vi "example test.vi"() -> ()   [LabVIEW 2013, in "io plugin tests.lvlib"]
uses:
  io plugin tests.lvlib
  module/configuration/tag bus configurable plugin module configuration.lvclass
  <vilib>/NI/Tag Bus Module Framework/channel/channel classification.ctl
  <vilib>/NI/Tag Bus/tag/Data Type.ctl
  module/execution/tag bus configurable plugin module.lvclass
  <vilib>/NI/Tag Bus/dictionary/data dictionary.lvclass/data dictionary.ctl
  <vilib>/NI/Tag Bus/dictionary/lookup polymorphs/locate double.vi
  <vilib>/NI/Tag Bus/table/data polymorphs/write one/write Double.vi
  <vilib>/NI/Tag Bus/table/data polymorphs/read one/read Double.vi
  <vilib>/NI/Tag Bus/dictionary/search/find data index.vi
  <vilib>/NI/Tag Bus/dictionary/search/search string list.vi
  <vilib>/NI/Tag Bus/dictionary/tag not found.vi
  <vilib>/NI/Tag Bus Module Framework/channel/TBM channel.lvclass
  <vilib>/NI/Tag Bus/tag/tag descriptor.lvclass
  <vilib>/NI/Tag Bus/dictionary/data dictionary.lvclass
  <vilib>/NI/Tag Bus/table/data table.lvlib
panel:
  out "final error":errorcluster
  out "output error":errorcluster
  out "input error":errorcluster
  out "output lookup error":errorcluster
  out "no data written":bool
  out "input lookup error":errorcluster
  out "init error":errorcluster
  out "correct execution settings":bool
  out "serialization problem":errorcluster
  out "invalid configuration":errorcluster
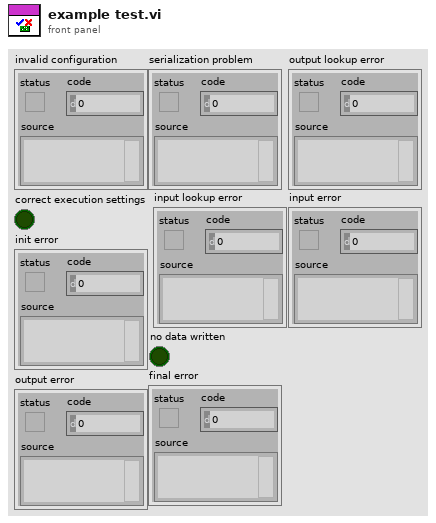
[diagram p1: front panel]
types:
  T1 = typedef "TBM channel.lvclass/channel classification.ctl" = enum16{"input data", "output data", "processing parameter", "processing result"}
  T2 = typedef "tag bus.lvlib/tag descriptor.lvclass/Data Type.ctl" = enum16{"Double", "Single", "I64", "I32", "I16", "I8", "U64", "U32", "U16", "U8", "Boolean", "String", "Array of Double", "Array of Single", "Array of I64", "Array of I32", "Array of I16", "Array of I8", "Array of U64", "Array of U32", "Array of U16", "Array of U8", "Array of Boolean", "Array of String"}
  T3 = typedef "TBM channel.lvclass/data tables.ctl" = cluster{"input data":T4, "processing parameter":T4, "processing result":T4, "output data":T4}
  T4 = typedef "tag bus.lvlib/dictionary table pair.ctl" = cluster{"data dictionary":refnum<class "data dictionary.lvclass">, "data table":T5}
  T5 = typedef "tag bus.lvlib/data table.lvlib/data table.ctl" = cluster{"Double":dbl[], "Single":sgl[], "I64":i64[], "I32":i32[], "I16":i16[], "I8":i8[], "U64":u64[], "U32":u32[], "U16":u16[], "U8":u8[], "Boolean":bool[], "String":string[], "Array of Double":cluster{"DBL Array":dbl[]}[], "Array of Single":cluster{"SGL Array":sgl[]}[], "Array of I64":cluster{"I64 Array":i64[]}[], "Array of I32":cluster{"I32 Array":i32[]}[], "Array of I16":cluster{"I16 Array":i16[]}[], "Array of I8":cluster{"I8 Array":i8[]}[], "Array of U64":cluster{"U64 Array":u64[]}[], "Array of U32":cluster{"U32 Array":u32[]}[], "Array of U16":cluster{"U16 Array":u16[]}[], "Array of U8":cluster{"U8 Array":u8[]}[], "Array of Boolean":cluster{"Boolean Array":bool[]}[], "Array of String":cluster{"String Array":string[]}[]}
  T6 = typedef "TBM module execution interface.lvclass/execution settings.ctl" = cluster{"reads inputs":bool, "processes data":bool, "writes outputs":bool}
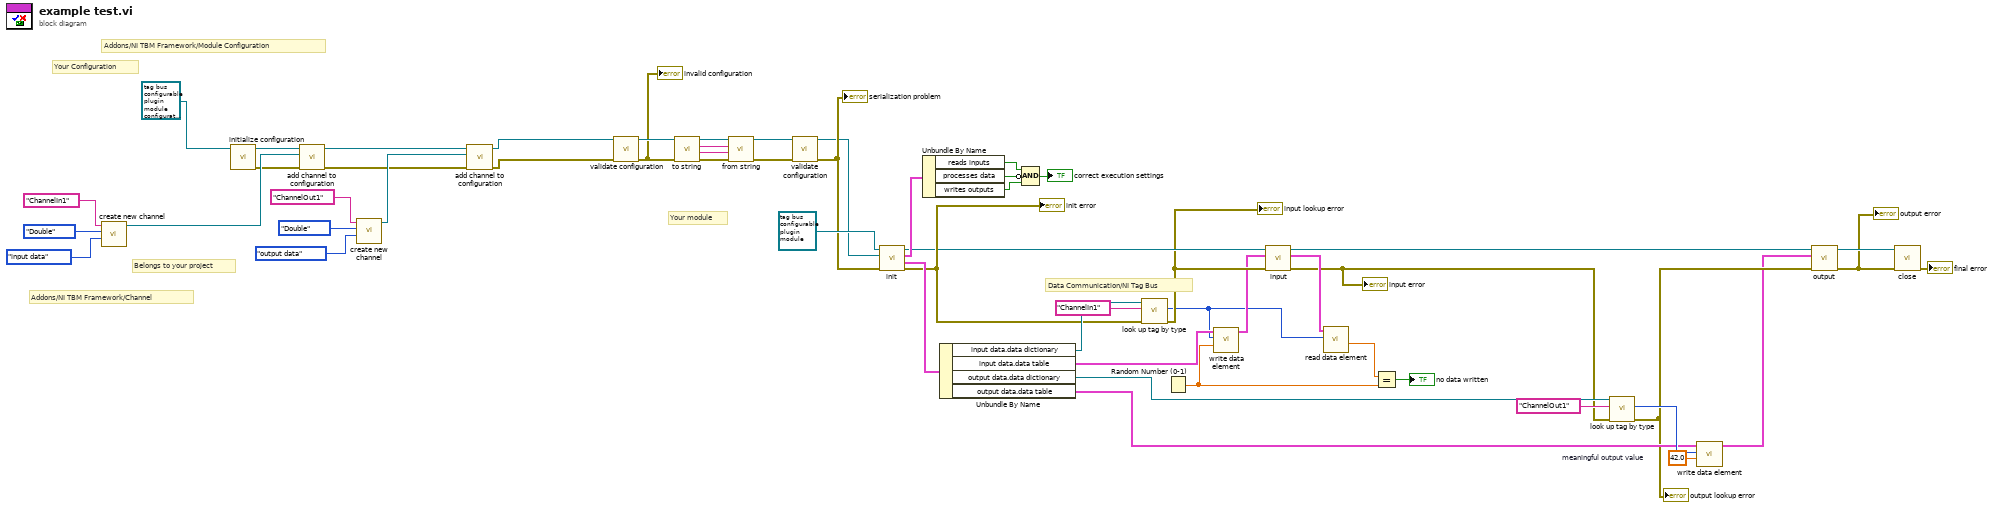
[diagram p0: block diagram]
diagram:
  w16 = 42.0  # meaningful output value
  # "Data Communication/NI Tag Bus"
  # "Your module"
  # "Your Configuration"
  # "Addons/NI TBM Framework/Module Configuration"
  # "Belongs to your project"
  # "Addons/NI TBM Framework/Channel"
  n1 = call <vilib>:"create new channel.vi"("channel classification"=channel_classification."input data", "data type"=Data_Type."Double", "channel name"="ChannelIn1") -> ("channel"=w5:refnum<class "TBM channel.lvclass">)  [unwired: 8 in]
  n2 = call-dynamic "initialize configuration.vi"("configuration in"=refnum<class "tag bus configurable plugin module configuration.lvclass"> refnum ("tag bus configurable plugin module configuration")) -> ("error out"=w2:errorcluster, "configuration out"=w3:refnum<class "tag bus configurable plugin module configuration.lvclass">)  [unwired: 8 in, 1 out]
  n3 = call "add channel to configuration.vi"("error in"=w2, "channel"=w5, "tag bus configurable plugin module configuration in"=w3) -> ("error out"=w4:errorcluster, "tag bus configurable plugin module configuration out"=w8:refnum<class "tag bus configurable plugin module configuration.lvclass">)  [unwired: 7 in]
  n4 = call <vilib>:"create new channel.vi"("channel classification"=channel_classification."output data", "data type"=Data_Type."Double", "channel name"="ChannelOut1") -> ("channel"=w6:refnum<class "TBM channel.lvclass">)  [unwired: 8 in]
  n5 = call "add channel to configuration.vi"("error in"=w4, "channel"=w6, "tag bus configurable plugin module configuration in"=w8) -> ("error out"=w1:errorcluster, "tag bus configurable plugin module configuration out"=w7:refnum<class "tag bus configurable plugin module configuration.lvclass">)  [unwired: 7 in]
  n6 = call-dynamic "validate configuration.vi"("error in"=w1, "tag bus configurable plugin module configuration in"=w7) -> ("error out"=w49:errorcluster, "tag bus configurable plugin module configuration out"=w50:refnum<class "tag bus configurable plugin module configuration.lvclass">)  [unwired: 8 in]
  "invalid configuration" <- w49
  n7 = call-dynamic "to string.vi"("error in"=w49, "tag bus configurable plugin module configuration in"=w50) -> ("error out"=w45:errorcluster, "data"=w46:string, "version"=w47:string, "tag bus configurable plugin module configuration out"=w48:refnum<class "tag bus configurable plugin module configuration.lvclass">)  [unwired: 6 in]
  n8 = call-dynamic "from string.vi"("error in"=w45, "data"=w46, "version"=w47, "tag bus configurable plugin module configuration in"=w48) -> ("error out"=w43:errorcluster, "tag bus configurable plugin module configuration out"=w44:refnum<class "tag bus configurable plugin module configuration.lvclass">)  [unwired: 6 in]
  n9 = call-dynamic "validate configuration.vi"("error in"=w43, "tag bus configurable plugin module configuration in"=w44) -> ("error out"=w41:errorcluster, "tag bus configurable plugin module configuration out"=w40:refnum<class "tag bus configurable plugin module configuration.lvclass">)  [unwired: 8 in]
  "serialization problem" <- w41
  n10 = call-dynamic "init.vi"("error in"=w41, "TBM module configuration in"=w40, "tag bus configurable plugin module in"=refnum<class "tag bus configurable plugin module.lvclass"> refnum ("tag bus configurable plugin module")) -> ("error out"=w32:errorcluster, "data allocations"=w34:T3, "execution settings"=w39:T6, "tag bus configurable plugin module out"=w29:refnum<class "tag bus configurable plugin module.lvclass">)  [unwired: 5 in]
  "init error" <- w32
  n11 = Unbundle By Name(w39) -> ("reads inputs"=w36:bool, "processes data"=w38:bool, "writes outputs"=w37:bool)
  n12 = Unbundle By Name(w34) -> ("input data.data dictionary"=w33:refnum<class "data dictionary.lvclass">, "input data.data table"=w30:T5, "output data.data dictionary"=w21:refnum<class "data dictionary.lvclass">, "output data.data table"=w18:T5)
  n13 = Compound Arithmetic op=AND(w36, invert w38, w37) -> (→"correct execution settings":bool)
  n14 = call-poly <vilib>:"look up tag by type.vi"("error in"=w32, "name"="ChannelIn1" ("channel name"), "data dictionary in"=w33) -> ("error out"=w28:errorcluster, "index"=w25:i32)  [unwired: 6 in, 1 out]
  "input lookup error" <- w28
  n15 = Random Number (0-1)() -> (number: 0 to 1=w24:dbl)
  n16 = call-poly <vilib>:"write data element.vi"("value"=w24, "index"=w25, "data table in"=w30) -> ("data table out"=w27:T5)  [unwired: 8 in]
  n17 = call-dynamic "input.vi"("error in"=w28, "data table in"=w27, "tag bus configurable plugin module in"=w29) -> ("error out"=w17:errorcluster, "data table out"=w26:T5, "tag bus configurable plugin module out"=w14:refnum<class "tag bus configurable plugin module.lvclass">)  [unwired: 6 in]
  "input error" <- w17
  n18 = call-poly <vilib>:"read data element.vi"("index"=w25, "data table in"=w26) -> ("value"=w23:dbl)  [unwired: 8 in, 1 out]
  n19 = Equal?(x=w23, y=w24) -> (x = y?=→"no data written":bool)
  n20 = call-poly <vilib>:"look up tag by type.vi"("error in"=w17, "name"="ChannelOut1" ("channel name"), "data dictionary in"=w21) -> ("error out"=w15:errorcluster, "index"=w19:i32)  [unwired: 6 in, 1 out]
  "output lookup error" <- w15
  n21 = call-poly <vilib>:"write data element.vi"("value"=w16, "index"=w19, "data table in"=w18) -> ("data table out"=w13:T5)  [unwired: 8 in]
  n22 = call-dynamic "output.vi"("error in"=w15, "data table in"=w13, "tag bus configurable plugin module in"=w14) -> ("error out"=w11:errorcluster, "tag bus configurable plugin module out"=w12:refnum<class "tag bus configurable plugin module.lvclass">)  [unwired: 6 in, 1 out]
  "output error" <- w11
  n23 = call-dynamic "close.vi"("error in"=w11, "tag bus configurable plugin module in"=w12) -> ("error out"=→"final error":errorcluster)  [unwired: 9 in]
